vi "List ARNs Recursive.vi"(8 "error in (no error)":errorcluster, 10 "NextToken":string, 11 "ARN in":refnum<class "ARN.lvclass">) -> (0 "error out":errorcluster, 3 "ARNs out":refnum<class "ARN.lvclass">[](array[class]))   [LabVIEW 2015, in "NI_AWS_Core.lvlib" / "ARN.lvclass"]
uses:
  ARN.lvclass
  HTTP Request/Request Options.ctl
  HTTP Request/Name Value Pair.ctl
  HTTP Request/HTTP Request.lvclass
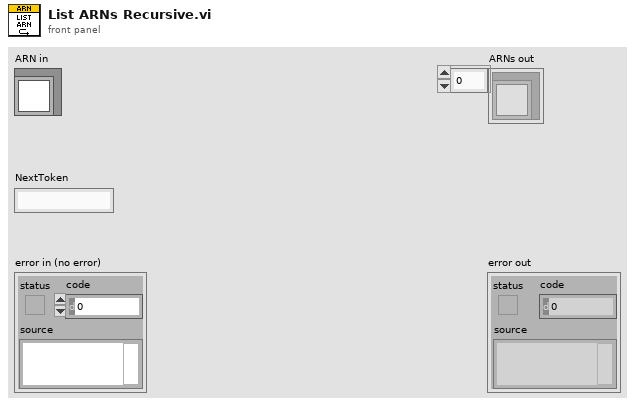
[diagram p1: front panel]
types:
  T1 = typedef "NI_AWS_Core.lvlib/HTTP Request.lvclass/Name Value Pair.ctl" = cluster{"name":string, "value":string}
  T2 = typedef "NI_AWS_Core.lvlib/HTTP Request.lvclass/Request Options.ctl" = cluster{"request headers":T1[], "request parameters":T1[], "request body":string, "ignore region":bool}
  T3 = typedef "NI_AWS_Core.lvlib/HTTP Request.lvclass/Response.ctl" = cluster{"Headers":string, "Body":string}
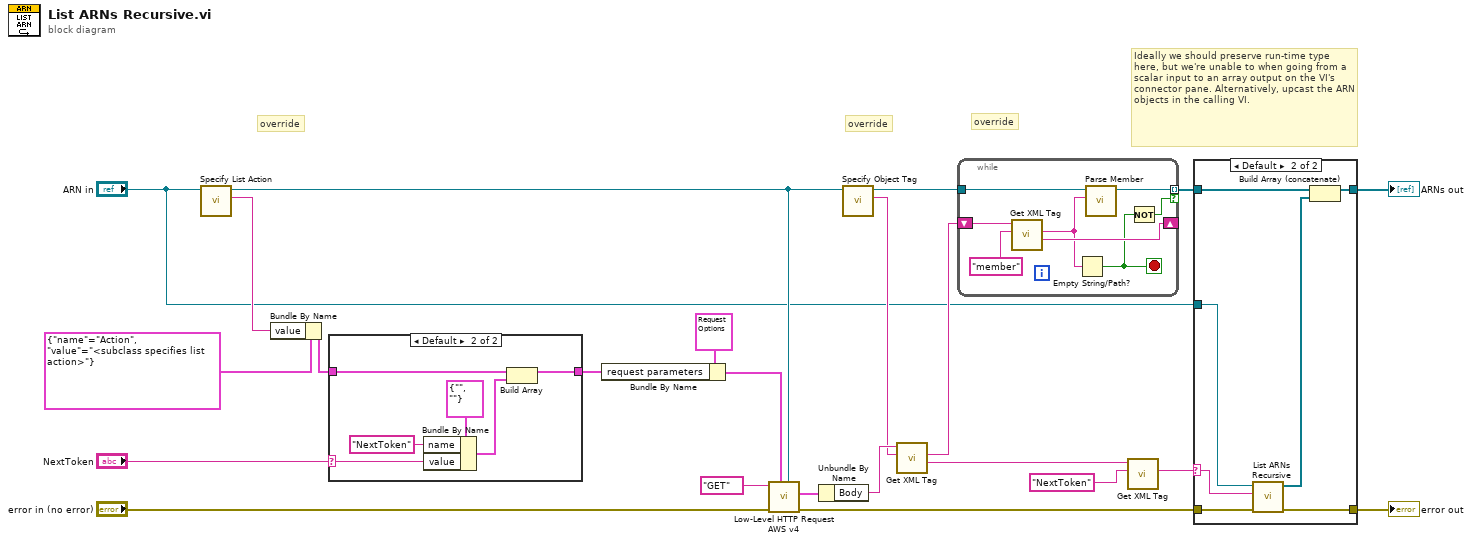
[diagram p0: block diagram]
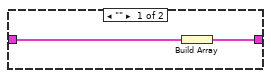
[diagram p3: hidden frame]
diagram:
  # "override"
  # "Ideally we should preserve run-time type here, but we're unable to when going from a scalar input to an array output on the VI's connector pane. Alternatively, upcast the ARN objects in the calling VI."
  # "override"
  # "override"
  n1 = call-dynamic "Specify List Action.vi"("ARN in"="ARN in") -> ("List Action"=w5:string, "ARN out"=w2:refnum<class "ARN.lvclass">)  [unwired: 9 in]
  n2 = Bundle By Name(cluster=T1 {"name"="Action", "value"="<subclass specifies list action>"} ("Cluster"), "value"=w5) -> (w6:T1)
  n3 = case shown="Default" "NextToken" {
    selector: "NextToken" -> [_ w26]
    tunnel: w6 -> [w25 w31]
    tunnel: [w24 w27] -> w16
    frame "" {
      n4 = Build Array(w25) -> (w24:T1[])
    }
    frame Default {
      n5 = Bundle By Name(cluster=T1 {"name"="", "value"=""} ("element"), "name"="NextToken", "value"=w26) -> (w28:T1)
      n6 = Build Array(w31, w28) -> (w27:T1[])
    }
  }
  n7 = Bundle By Name(cluster=T2 {"request headers"=[], "request parameters"=[{"name"="Action", "value"="ListQueues"}], "request body"="", "ignore region"=FALSE} ("Request Options"), "request parameters"=w16) -> (w20:T2)
  n8 = call "Low-Level HTTP Request AWS v4.vi"("AWS Core"=w2, "Request Options"=w20, "error in (no error)"="error in (no error)", "HTTP-Verb"="GET") -> ("error out"=w15:errorcluster, "Response"=w19:T3)  [unwired: 5 in, 1 out]
  n9 = Unbundle By Name(w19) -> ("Body"=w10:string)
  n10 = call-dynamic "Specify Object Tag.vi"("ARN in"=w2) -> ("Object tag"=w3:string, "ARN out"=w4:refnum<class "ARN.lvclass">)  [unwired: 9 in]
  n11 = call "Get XML Tag.vi"("Tag name"=w3, "XML String in"=w10) -> ("Remaining string"=w9:string, "Tag value"=w11:string)  [unwired: 5 in, 3 out]
  n12 = while {
    shift-right: [w38] -> _
    shift-left: w11 -> [w39]
    tunnel: w4 -> [w34]
    tunnel: [w33] -> w8 mode=indexing if=w35
    stop <- w36 stop-if-true
    n13 = call "Get XML Tag.vi"("Tag name"="member", "XML String in"=w39) -> ("Remaining string"=w38:string, "Tag value"=w32:string)  [unwired: 5 in, 3 out]
    n14 = Empty String/Path?(string/path=w32) -> (empty?=w36:bool)
    n15 = call-dynamic "Parse Member.vi"("member"=w32, "ARN in"=w34) -> ("ARN out"=w33:refnum<class "ARN.lvclass">)  [unwired: 8 in, 1 out]
    n16 = Not(x=w36) -> (.not. x?=w35:bool)
  }
  n17 = call "Get XML Tag.vi"("Tag name"="NextToken", "XML String in"=w9) -> ("Tag value"=w13:string)  [unwired: 5 in, 4 out]
  n18 = case shown="Default" w13 {
    selector: w13 -> [_ w43]
    tunnel: w15 -> [w41 w48]
    tunnel: [w41 w47] -> w14
    tunnel: w8 -> [w40 w46]
    tunnel: [w40 w44] -> w12
    tunnel: "ARN in" -> [_ w42]
    frame "" {
    }
    frame Default {
      n19 = call "List ARNs Recursive.vi"("error in (no error)"=w48, "NextToken"=w43, "ARN in"=w42) -> ("error out"=w47:errorcluster, "ARNs out"=w45:refnum<class "ARN.lvclass">[])  [unwired: 7 in]
      n20 = Build Array (concatenate)(w46, w45) -> (w44:refnum<class "ARN.lvclass">[])
    }
  }
  "error out" <- w14
  "ARNs out" <- w12
